vi "Remove Active Object.vi"(11 "Core Data in":T1) -> (3 "Core Data out":T1)   [LabVIEW 2020, in "Amnesia.lvlib"]
uses:
  Amnesia.lvlib
  Scene/Scene.lvclass
  Core Data.ctl
  Scene/Mouse Button Held.ctl
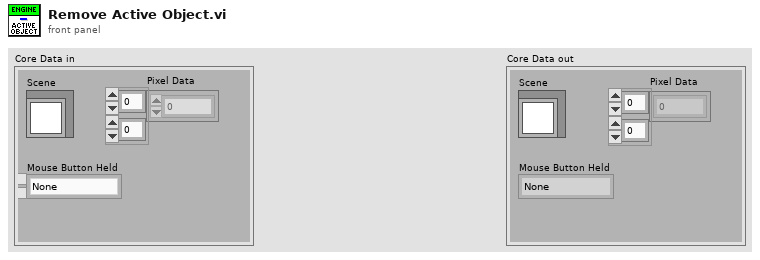
[diagram p1: front panel]
types:
  T1 = typedef "Amnesia.lvlib/Core Data.ctl" = cluster{"Pixel Data":u32[][], "Scene":refnum<class "Scene.lvclass">, "Mouse Button Held":T2}
  T2 = typedef "Scene.lvclass/Mouse Button Held.ctl" = enum16{"None", "Left", "Middle", "Right"}
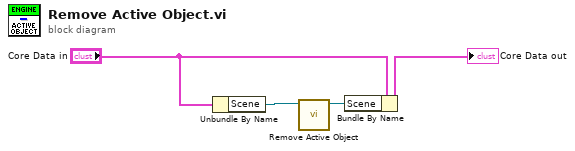
[diagram p0: block diagram]
diagram:
  n1 = Unbundle By Name("Core Data in") -> ("Scene"=w2:refnum<class "Scene.lvclass">)
  n2 = call "Remove Active Object.vi"("Scene in"=w2) -> ("Scene out"=w1:refnum<class "Scene.lvclass">)  [unwired: 10 in]
  n3 = Bundle By Name(cluster="Core Data in", "Scene"=w1) -> (→"Core Data out":T1)
